vi "CheckForEmptyPath.vi"(8 "error in (no error)":errorcluster, 11 "file path in":path) -> (0 "error out":errorcluster, 3 "file path in":path)   [LabVIEW 2025]
uses:
  <vilib>/measure/NI_MABase.lvlib
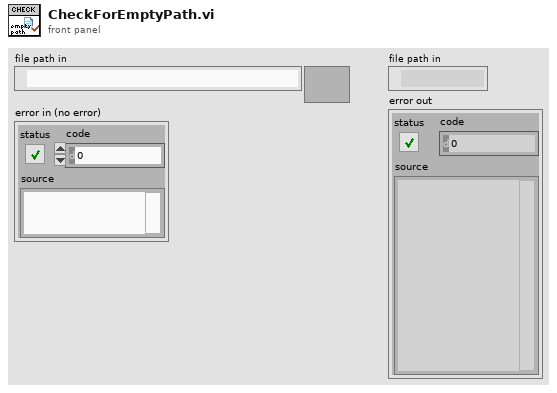
[diagram p1: front panel]
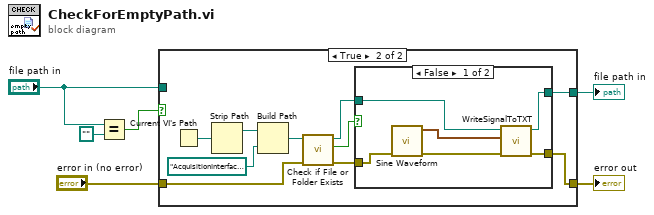
[diagram p0: block diagram]
diagram:
  n1 = Equal?(x="file path in", y=path "") -> (x = y?=w5:bool)
  n2 = case shown="True" w5 {
    tunnel: [w8 w16] -> w3
    tunnel: "file path in" -> [w8 _]
    tunnel: "error in (no error)" -> [w7 w18]
    tunnel: [w7 w14] -> w1
    frame False {
    }
    frame True {
      n3 = Current VI's Path() -> (path=w13:path)
      n4 = Strip Path(path=w13) -> (stripped path=w12:path)  [unwired: 1 out]
      n5 = Build Path(base path=w12, name or relative path=path "AcquisitionInterface2-files/signal.txt") -> (appended path=w10:path)
      n6 = call <vilib>:"Check if File or Folder Exists.vi"("error in (no error)"=w18, "path"=w10) -> ("error out"=w15:errorcluster, "file or folder exists?"=w9:bool, "dup path"=w17:path)  [unwired: 7 in]
      n7 = case shown="False" w9 {
        tunnel: [w20 w26] -> w16
        tunnel: w17 -> [w22 w26]
        tunnel: w15 -> [w21 w25]
        tunnel: [w19 w25] -> w14
        frame False {
          n8 = call <vilib>:"Sine Waveform.vi"("error in (no error)"=w21) -> ("error out"=w23:errorcluster, "signal out"=w24:waveform(dbl))  [unwired: 9 in]
          n9 = call "WriteSignalToTXT.vi"("error in"=w23, "waveform"=w24, "file path in"=w22) -> ("error out"=w19:errorcluster, "file path out"=w20:path)  [unwired: 7 in]
        }
        frame True {
        }
      }
    }
  }
  "file path in" <- w3
  "error out" <- w1
